vi "GetStructMembersAsNameAndValue.vi"(8 "error in (no error)":errorcluster, 11 "Struct Parameter":string="<value><struct><member><name>two</name><value><i4>2</i4></value></member><member><name>one</name><value><i4>1</i4></value></member><member><name>three</name><value><i4>3</i4></value></member></struct></value>") -> (0 "error out":errorcluster, 3 "struct members":T1[](array[typedef]))   [LabVIEW 2009]
doc: "Unpack XML-RPC struct into LV name/value pairs (strings)"
uses:
  XML-RPC Message Builder/struct/structMember.ctl
panel:
  in  "member (data prototype)":T1
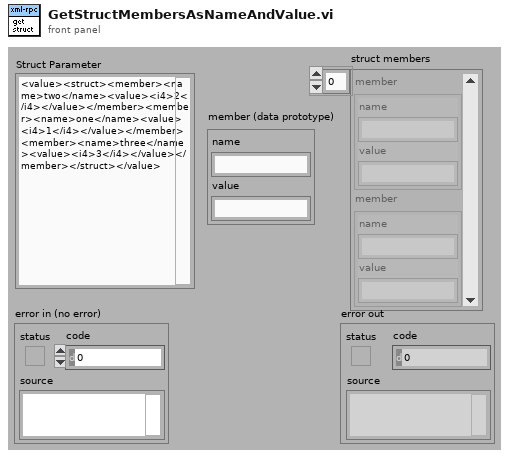
[diagram p1: front panel]
types:
  T1 = typedef "structMember.ctl" = cluster{"name":string, "value":string}
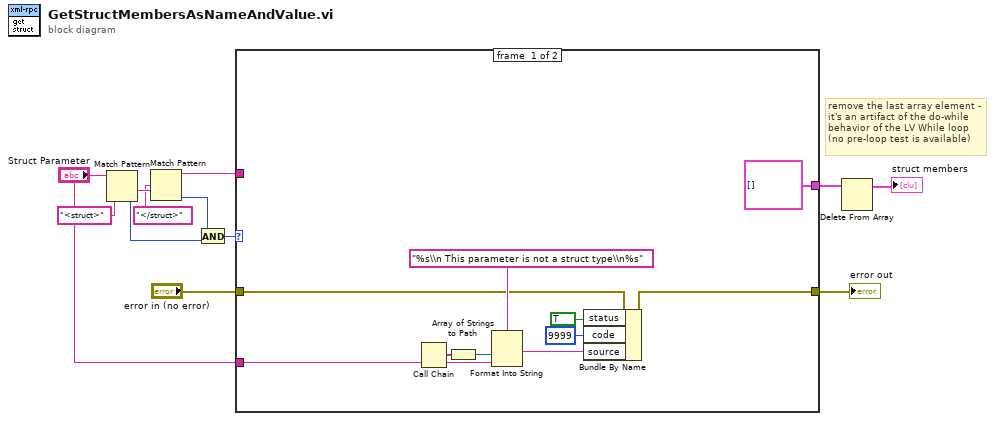
[diagram p0: block diagram]
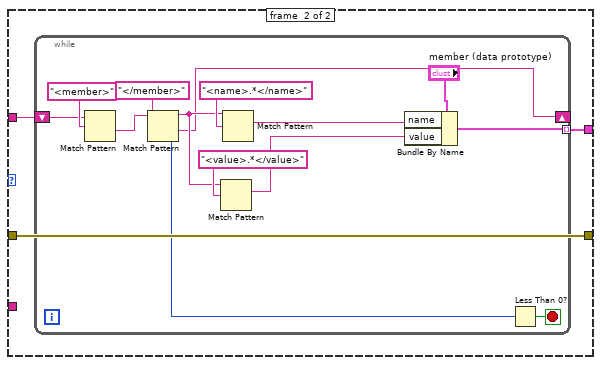
[diagram p2: hidden frame]
diagram:
  # "remove the last array element - it's an artifact of the do-while behavior of the LV While loop (no pre-loop test is available)"
  n1 = Match Pattern(string="Struct Parameter", regular expression="<struct>") -> (after substring=w11:string, offset past match=w8:i32)  [unwired: 1 in, 2 out]
  n2 = Match Pattern(string=w11, regular expression="</struct>") -> (before substring=w6:string, offset past match=w9:i32)  [unwired: 1 in, 2 out]
  n3 = And(x=w9, y=w8) -> (x .and. y?=w7:i32)
  n4 = case shown="-1" w7 {
    tunnel: w6 -> [_ w25]
    tunnel: [T1[] [] w24] -> w5
    tunnel: "error in (no error)" -> [w15 w23]
    tunnel: [w14 w23] -> w2
    tunnel: "Struct Parameter" -> [w13 _]
    frame #0 {
      n5 = Call Chain() -> (call chain=w16:string[])
      n6 = Array of Strings to Path(0:w16) -> (2:w19:path)  [unwired: 1 in]
      n7 = Format Into String(format string="%s\\n This parameter is not a struct type\\n%s", w19, w13) -> (resulting string=w20:string)  [unwired: 2 in, 1 out]
      n8 = Bundle By Name(cluster=w15, "status"=TRUE, "code"=9999, "source"=w20) -> (w14:errorcluster)
    }
    frame #1 {
      n9 = while {
        tunnel: [w28] -> w24 mode=indexing
        shift-right: [w26] -> _
        shift-left: w25 -> [w36]
        stop <- w34 stop-if-true
        n10 = Match Pattern(string=w36, regular expression="<member>") -> (after substring=w37:string)  [unwired: 1 in, 3 out]
        n11 = Match Pattern(string=w37, regular expression="</member>") -> (before substring=w27:string, after substring=w26:string, offset past match=w35:i32)  [unwired: 1 in, 1 out]
        n12 = Match Pattern(string=w27, regular expression="<value>.*</value>") -> (match substring=w29:string)  [unwired: 1 in, 3 out]
        n13 = Match Pattern(string=w27, regular expression="<name>.*</name>") -> (match substring=w30:string)  [unwired: 1 in, 3 out]
        n14 = Bundle By Name(cluster="member (data prototype)", "name"=w30, "value"=w29) -> (w28:T1)
        n15 = Less Than 0?(x=w35) -> (x < 0?=w34:bool)
      }
    }
  }
  "error out" <- w2
  n16 = Delete From Array(array=w5) -> (array with subset deleted=→"struct members":T1[])  [unwired: 2 in, 1 out]
